vi "Renishaw-XL80_GetMl10Status.vi"(8 "error in (no error)":errorcluster, 11 "Renishaw-XL80 in":refnum<class "Renishaw-XL80.lvclass">) -> (0 "error out":errorcluster, 2 "ML10Status":i32(ring)=1 items=["ML10_AVERAGING_ON"=1, "ML10_TPIN_SELECTED"=4, "ML10_BEAM_LOW"=64, "ML10_BEAM_LOSS"=128, "ML10_STABILITY_LOSS"=256, "ML10_PREHEAT"=2048, "ML10_LASER_TOO_COLD"=4096, "ML10_LASER_TOO_HOT"=8192, "ML10_LASER_UNSTABLE"=16384, "ML10_LASER_FAIL"=32768, "ML10_NOT_RESPONDING"=65536, "ML10_LONG_TERM_AVERAGING_ON"=524288, "ML10_MEASUREMENT_MODE"=7340032, "ML10_HIGH_SPEED_ERROR"=8388608, "ML10_DYNAMIC_SELECTED"=16777216], 3 "Renishaw-XL80 out":refnum<class "Renishaw-XL80.lvclass">)   [LabVIEW 2024, in "Renishaw-XL80.lvclass"]
doc: "This read only property returns the current status of the ML10.\n\nDefinition\nHRESULTget_ML10Status( [out, retval] ML10_STATUS_CODES* pVal);\nParameters\npVal\nA variable that will be set to ML10_STATUS_CODES.\n\nComments\nThis property will return with an HRESULT of E_FAIL if the client has not previously connected to a DX10 by calling Connect.\n\nIf the client has connected then this property will normally return an HRESULT of S_OK. However, it will return E_POINTER if the client supplies a null pointer for pVal.\n\nNote: if there is a XL laser connected to the DX10Adaptor COM interface then this property returns the XL laser's status"
uses:
  Renishaw-XL80.lvclass
  Renishaw-XL80.lvclass/Renishaw-XL80.ctl
  D:/A.C.M/Example CSharp_64/bin/Debug/Interop.DX10SDKADAPTORLib.dll
  Example CSharp_64/bin/Debug/Interop.DX10SDKADAPTORLib.dll
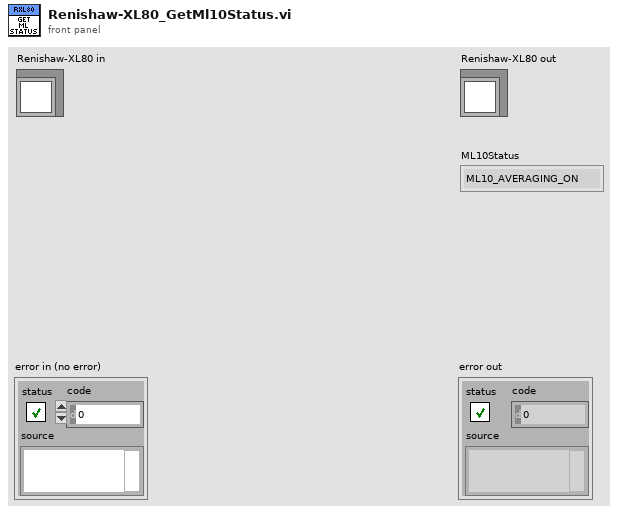
[diagram p1: front panel]
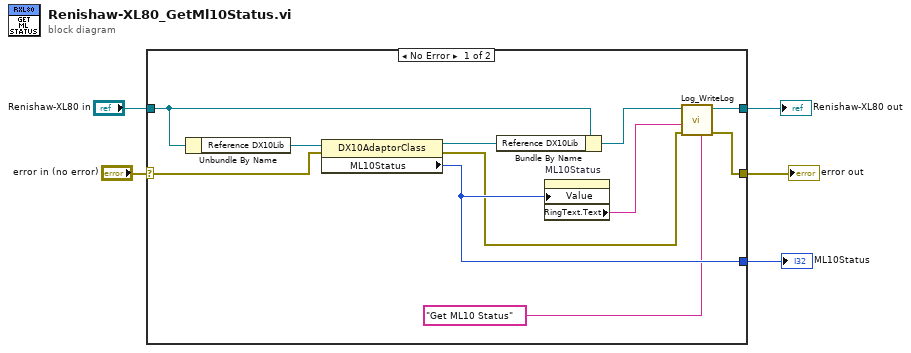
[diagram p0: block diagram]
diagram:
  n1 = case shown="No Error" "error in (no error)" {
    selector: "error in (no error)" -> [w13 w18]
    tunnel: [w11 w18] -> w4
    tunnel: [w12 w17] -> w2
    tunnel: "Renishaw-XL80 in" -> [w14 w17]
    tunnel: [w9 _] -> w1
    frame No Error {
      n2 = Unbundle By Name(w14) -> ("Reference DX10Lib"=w16:refnum<k24>)
      n3 = property class="DX10AdaptorClass"(reference=w16, error in=w13) -> (reference out=w15:refnum<k24>, error out=w6:errorcluster, "ML10Status"=w9:i32)
      n4 = Bundle By Name(cluster=w14, "Reference DX10Lib"=w15) -> (w10:refnum<class "Renishaw-XL80.lvclass">)
      n5 = property on="ML10Status" class="Ring (strict)"("Value"=w9) -> ("RingText.Text"=w8:string)  [unwired: 2 in, 2 out]
      n6 = call-dynamic "Log_WriteLog.vi"("Additional text"="Get ML10 Status", "error in (no error)"=w6, "Response"=w8, "Log in"=w10) -> ("error out"=w11:errorcluster, "Log out"=w12:refnum<class "Renishaw-XL80.lvclass">)  [unwired: 6 in]
    }
    frame Error {
    }
  }
  "error out" <- w4
  "Renishaw-XL80 out" <- w2
  "ML10Status" <- w1
